vi "Configure Measurements Number.vi"(8 "error in (no error)":errorcluster, 10 "Measurements Points (1)":i32=1, 11 "VISA resource name":refnum<visa-resource-name>) -> (0 "error out":errorcluster, 3 "VISA resource name out":refnum<visa-resource-name>)   [LabVIEW 2018, in "Agilent U2000 Series.lvlib"]
doc: "Sets the number of measurements to be made.\n\nNote: \n(1) This VI is only applicable for U2040 X-Series.\n(2) The number of measurement points can be calculated using the following equation:\nPoints = (|Stop frequency - Start frequency|/Frequency step)+ 1 while both of the start and stop frequency can be set in <b>Configure Frequency Sweep List.vi</b>"
uses:
  Agilent U2000 Series.lvlib
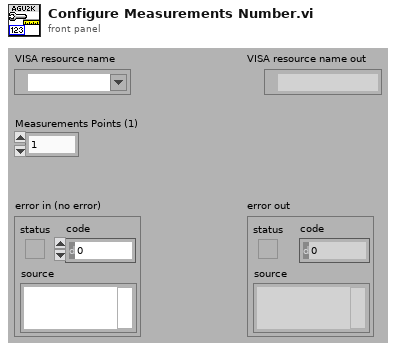
[diagram p1: front panel]
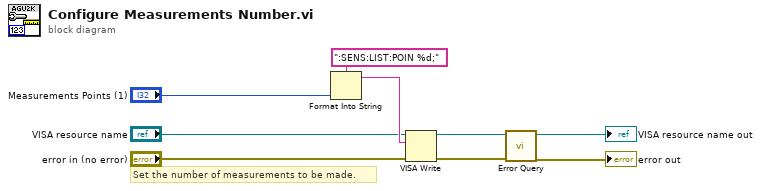
[diagram p0: block diagram]
diagram:
  # "Set the number of measurements to be made."
  n1 = Format Into String(format string=":SENS:LIST:POIN %d;", "Measurements Points (1)") -> (resulting string=w7:string)  [unwired: 2 in, 1 out]
  n2 = VISA Write(VISA resource name="VISA resource name", write buffer=w7, error in (no error)="error in (no error)") -> (VISA resource name out=w4:refnum<visa-resource-name>, error out=w3:errorcluster)  [unwired: 1 out]
  n3 = call "Error Query.vi"("error in (no error)"=w3, "VISA resource name"=w4) -> ("error out"=→"error out":errorcluster, "VISA resource name out"=→"VISA resource name out":refnum<visa-resource-name>)  [unwired: 6 in, 2 out]
